vi "test Loopback MC with Start and Stop.vi"(8 "error in":errorcluster, 11 "TestCase in":refnum<class "Loopback.lvclass">) -> (0 "error out":errorcluster, 3 "TestCase out":refnum<class "Loopback.lvclass">)   [LabVIEW 2020, in "Loopback.lvclass"]
uses:
  Loopback.lvclass
  C:/dev/niveristand-custom-device-testing-tools/VeriStandTestCase/VeriStandTestCase.lvclass
  <vilib>/numeric/Random Number (Range) U64.vi
  485b7c2b-8320-4722-9ec7-d01f27c65546.vi
  cbc5c385-99ae-4ee9-9433-d6a44dd842bc.vi
  412f3c08-5d5c-44d4-ba0c-e78ba60fad11.vi
  849d8f76-503e-4f73-a17f-6140b744aaa7.vi
  0f9dda61-2c21-4955-8588-a8fc95227647.vi
  c1072d6c-53a2-4b9a-88af-ad4a91435edd.vi
  d6433e8a-b9d0-4f33-89c0-bfe3ca19b651.vi
  62366d90-b7ce-4d5b-90d7-fbdeef7ff138.vi
  <vilib>/numeric/sub_Random U32.vi
  <vilib>/NI VeriStand/Execution/Workspace/NI VeriStand - Set Single Channel Value.vi
  <vilib>/NI VeriStand/Execution/Workspace/NI VeriStand - Get Single Channel Value.vi
  <vilib>/addons/_JKI Toolkits/VI Tester/TestCase.llb/TestCase.lvclass
  <vilib>/NI VeriStand/Execution/Workspace/NI_VS Workspace ExecutionAPI.lvlib
  C:/Program Files (x86)/National Instruments/LabVIEW 2020/vi.lib/addons/_JKI Toolkits/VI Tester/TestCase.llb/TestCase.lvclass
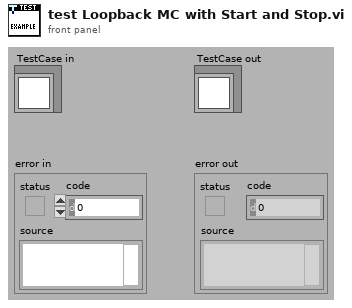
[diagram p1: front panel]
types:
  T1 = typedef "NI_VS Workspace ExecutionAPI.lvlib/WorkspaceAPI.ctl" = refnum<k24>
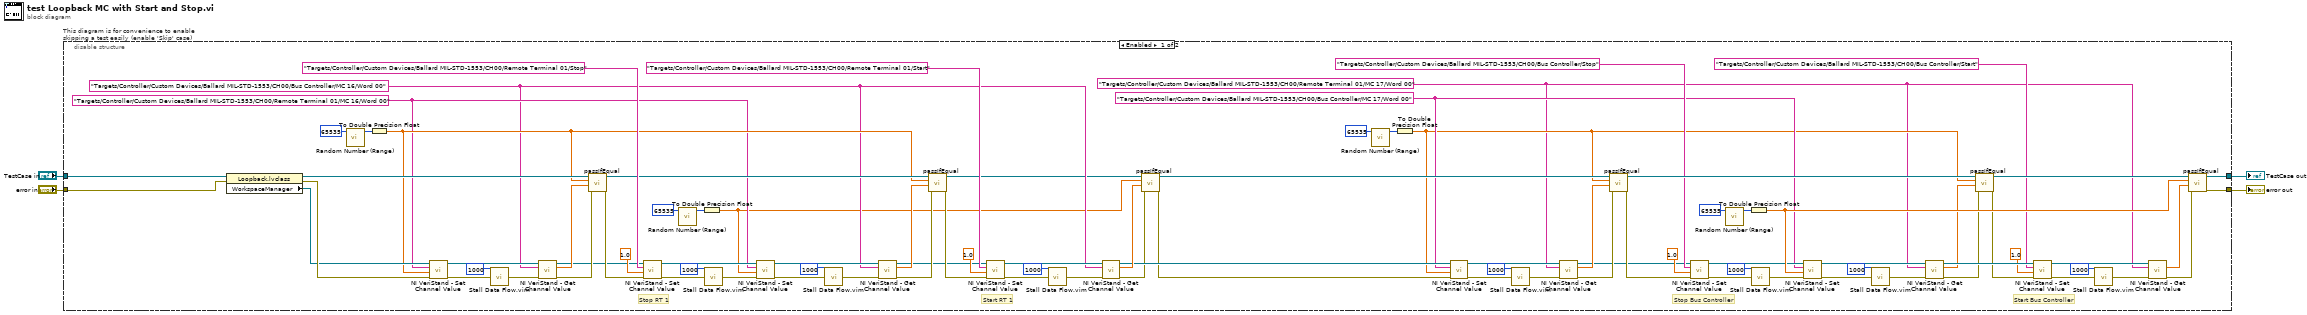
[diagram p0: block diagram]
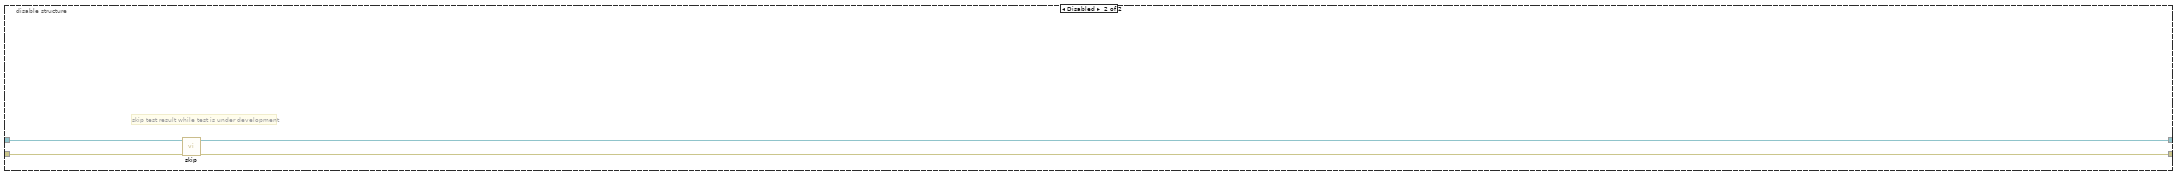
[diagram p2: hidden frame]
diagram:
  n1 = disable-structure "This diagram is for convenience to enable skipping a test easily (enable 'Skip' case)" shown="Enabled" {
    disable-tunnel: "TestCase in" -> [w85 w98]
    disable-tunnel: [w7 w96] -> w1
    disable-tunnel: [w6 w97] -> w3
    disable-tunnel: "error in" -> [w84 w95]
    frame Enabled {
      w8 = "Targets/Controller/Custom Devices/Ballard MIL-STD-1553/CH00/Remote Terminal 01/MC 17/Word 00" ("Channel")
      w11 = "Targets/Controller/Custom Devices/Ballard MIL-STD-1553/CH00/Bus Controller/MC 17/Word 00" ("Channel")
      w47 = "Targets/Controller/Custom Devices/Ballard MIL-STD-1553/CH00/Bus Controller/MC 16/Word 00" ("Channel")
      w61 = "Targets/Controller/Custom Devices/Ballard MIL-STD-1553/CH00/Remote Terminal 01/MC 16/Word 00" ("Channel")
      # "Start Bus Controller"
      # "Stop Bus Controller"
      # "Start RT 1"
      # "Stop RT 1"
      n2 = property class="Loopback.lvclass"(reference=w85, error in=w84) -> (reference out=w94:refnum<class "Loopback.lvclass">, error out=w89:errorcluster, "WorkspaceManager"=w87:T1)
      n3 = call-poly <vilib>:"Random Number (Range).vi"("upper bound (100)"=u64 65535) -> ("number"=w77:u64)  [unwired: 10 in]
      n4 = To Double Precision Float(number=w77) -> (double precision float=w65:dbl)
      n5 = call-poly <vilib>:"NI VeriStand - Set Channel Value.vi"("error in (no error)"=w89, "Value"=w65, "Channel"=w61, "WorkspaceManager in"=w87) -> ("error out"=w91:errorcluster, "WorkspaceManager out"=w93:T1)  [unwired: 6 in]
      n6 = call "Stall Data Flow.vim"("value in"=w91, "milliseconds to wait"=u32 1000) -> ("value out"=w92:errorcluster)  [unwired: 1 out]
      n7 = call-poly <vilib>:"NI VeriStand - Get Channel Value.vi"("error in (no error)"=w92, "Channel"=w47, "WorkspaceManager in"=w93) -> ("error out"=w88:errorcluster, "Value"=w86:dbl, "WorkspaceManager out"=w39:T1)  [unwired: 6 in]
      n8 = call-dynamic "passIfEqual.vi"("error in (no error)"=w88, "y"=w86, "x"=w65, "TestCase in"=w94) -> ("error out"=w69:errorcluster, "TestCase out"=w66:refnum<class "Loopback.lvclass">)  [unwired: 6 in]
      n9 = call-poly <vilib>:"NI VeriStand - Set Channel Value.vi"("error in (no error)"=w69, "Value"=1.0, "Channel"="Targets/Controller/Custom Devices/Ballard MIL-STD-1553/CH00/Remote Terminal 01/Stop", "WorkspaceManager in"=w39) -> ("error out"=w70:errorcluster, "WorkspaceManager out"=w63:T1)  [unwired: 6 in]
      n10 = call-poly <vilib>:"Random Number (Range).vi"("upper bound (100)"=u64 65535) -> ("number"=w56:u64)  [unwired: 10 in]
      n11 = To Double Precision Float(number=w56) -> (double precision float=w44:dbl)
      n12 = call "Stall Data Flow.vim"("value in"=w70, "milliseconds to wait"=u32 1000) -> ("value out"=w64:errorcluster)  [unwired: 1 out]
      n13 = call-poly <vilib>:"NI VeriStand - Set Channel Value.vi"("error in (no error)"=w64, "Value"=w44, "Channel"=w61, "WorkspaceManager in"=w63) -> ("error out"=w59:errorcluster, "WorkspaceManager out"=w62:T1)  [unwired: 6 in]
      n14 = call "Stall Data Flow.vim"("value in"=w59, "milliseconds to wait"=u32 1000) -> ("value out"=w58:errorcluster)  [unwired: 1 out]
      n15 = call-poly <vilib>:"NI VeriStand - Get Channel Value.vi"("error in (no error)"=w58, "Channel"=w47, "WorkspaceManager in"=w62) -> ("error out"=w72:errorcluster, "Value"=w73:dbl, "WorkspaceManager out"=w50:T1)  [unwired: 6 in]
      n16 = call-dynamic "passIfEqual.vi"("error in (no error)"=w72, "y"=w73, "x"=w65, "TestCase in"=w66) -> ("error out"=w52:errorcluster, "TestCase out"=w46:refnum<class "Loopback.lvclass">)  [unwired: 6 in]
      n17 = call-poly <vilib>:"NI VeriStand - Set Channel Value.vi"("error in (no error)"=w52, "Value"=1.0, "Channel"="Targets/Controller/Custom Devices/Ballard MIL-STD-1553/CH00/Remote Terminal 01/Start", "WorkspaceManager in"=w50) -> ("error out"=w54:errorcluster, "WorkspaceManager out"=w49:T1)  [unwired: 6 in]
      n18 = call "Stall Data Flow.vim"("value in"=w54, "milliseconds to wait"=u32 1000) -> ("value out"=w48:errorcluster)  [unwired: 1 out]
      n19 = call-poly <vilib>:"NI VeriStand - Get Channel Value.vi"("error in (no error)"=w48, "Channel"=w47, "WorkspaceManager in"=w49) -> ("error out"=w42:errorcluster, "Value"=w45:dbl, "WorkspaceManager out"=w43:T1)  [unwired: 6 in]
      n20 = call-dynamic "passIfEqual.vi"("error in (no error)"=w42, "y"=w45, "x"=w44, "TestCase in"=w46) -> ("error out"=w41:errorcluster, "TestCase out"=w40:refnum<class "Loopback.lvclass">)  [unwired: 6 in]
      n21 = call-poly <vilib>:"Random Number (Range).vi"("upper bound (100)"=u64 65535) -> ("number"=w75:u64)  [unwired: 10 in]
      n22 = To Double Precision Float(number=w75) -> (double precision float=w10:dbl)
      n23 = call-poly <vilib>:"NI VeriStand - Set Channel Value.vi"("error in (no error)"=w41, "Value"=w10, "Channel"=w11, "WorkspaceManager in"=w43) -> ("error out"=w80:errorcluster, "WorkspaceManager out"=w78:T1)  [unwired: 6 in]
      n24 = call "Stall Data Flow.vim"("value in"=w80, "milliseconds to wait"=u32 1000) -> ("value out"=w79:errorcluster)  [unwired: 1 out]
      n25 = call-poly <vilib>:"NI VeriStand - Get Channel Value.vi"("error in (no error)"=w79, "Channel"=w8, "WorkspaceManager in"=w78) -> ("error out"=w82:errorcluster, "Value"=w83:dbl, "WorkspaceManager out"=w5:T1)  [unwired: 6 in]
      n26 = call-dynamic "passIfEqual.vi"("error in (no error)"=w82, "y"=w83, "x"=w10, "TestCase in"=w40) -> ("error out"=w14:errorcluster, "TestCase out"=w13:refnum<class "Loopback.lvclass">)  [unwired: 6 in]
      n27 = call-poly <vilib>:"NI VeriStand - Set Channel Value.vi"("error in (no error)"=w14, "Value"=1.0, "Channel"="Targets/Controller/Custom Devices/Ballard MIL-STD-1553/CH00/Bus Controller/Stop", "WorkspaceManager in"=w5) -> ("error out"=w18:errorcluster, "WorkspaceManager out"=w21:T1)  [unwired: 6 in]
      n28 = call-poly <vilib>:"Random Number (Range).vi"("upper bound (100)"=u64 65535) -> ("number"=w27:u64)  [unwired: 10 in]
      n29 = To Double Precision Float(number=w27) -> (double precision float=w37:dbl)
      n30 = call "Stall Data Flow.vim"("value in"=w18, "milliseconds to wait"=u32 1000) -> ("value out"=w20:errorcluster)  [unwired: 1 out]
      n31 = call-poly <vilib>:"NI VeriStand - Set Channel Value.vi"("error in (no error)"=w20, "Value"=w37, "Channel"=w11, "WorkspaceManager in"=w21) -> ("error out"=w24:errorcluster, "WorkspaceManager out"=w22:T1)  [unwired: 6 in]
      n32 = call "Stall Data Flow.vim"("value in"=w24, "milliseconds to wait"=u32 1000) -> ("value out"=w25:errorcluster)  [unwired: 1 out]
      n33 = call-poly <vilib>:"NI VeriStand - Get Channel Value.vi"("error in (no error)"=w25, "Channel"=w8, "WorkspaceManager in"=w22) -> ("error out"=w16:errorcluster, "Value"=w15:dbl, "WorkspaceManager out"=w32:T1)  [unwired: 6 in]
      n34 = call-dynamic "passIfEqual.vi"("error in (no error)"=w16, "y"=w15, "x"=w10, "TestCase in"=w13) -> ("error out"=w31:errorcluster, "TestCase out"=w35:refnum<class "Loopback.lvclass">)  [unwired: 6 in]
      n35 = call-poly <vilib>:"NI VeriStand - Set Channel Value.vi"("error in (no error)"=w31, "Value"=1.0, "Channel"="Targets/Controller/Custom Devices/Ballard MIL-STD-1553/CH00/Bus Controller/Start", "WorkspaceManager in"=w32) -> ("error out"=w29:errorcluster, "WorkspaceManager out"=w33:T1)  [unwired: 6 in]
      n36 = call "Stall Data Flow.vim"("value in"=w29, "milliseconds to wait"=u32 1000) -> ("value out"=w34:errorcluster)  [unwired: 1 out]
      n37 = call-poly <vilib>:"NI VeriStand - Get Channel Value.vi"("error in (no error)"=w34, "Channel"=w8, "WorkspaceManager in"=w33) -> ("error out"=w38:errorcluster, "Value"=w36:dbl)  [unwired: 6 in, 1 out]
      n38 = call-dynamic "passIfEqual.vi"("error in (no error)"=w38, "y"=w36, "x"=w37, "TestCase in"=w35) -> ("error out"=w6:errorcluster, "TestCase out"=w7:refnum<class "Loopback.lvclass">)  [unwired: 6 in]
    }
    frame Disabled {
      # "skip test result while test is under development"
      n39 = call <vilib>:"skip.vi"("error in (no error)"=w95, "TestCase in"=w98) -> ("error out"=w97:errorcluster, "TestCase out"=w96:refnum<class "Loopback.lvclass">)  [unwired: 8 in]
    }
  }
  "error out" <- w3
  "TestCase out" <- w1
